vi "Module Execution Main.vi"() -> ()   [LabVIEW 2013, in "module execution process.lvlib"]
uses:
  module execution process.lvlib
  SubVIs/queue name.ctl
  SubVIs/command commands to rtexe process.ctl
  <vilib>/NI/Module Execution Interface/Engine Runtime/Engine Runtime Interface.lvclass
  <vilib>/NI/Configuration Framework/class discovery singleton/class discovery singleton methods.ctl
  <vilib>/NI/Tag Bus Data Framework/Framework Configuration Classes/target runtime/PL_Target Runtime.lvclass
  SubVIs/engine status data.ctl
  <vilib>/NI/Module Execution Interface/Engine Runtime/Execution States.ctl
  <vilib>/NI/AMC/Read Termination Message.vi
  <vilib>/NI/AMC/Create Single Message.vi
  <vilib>/NI/AMC/Globals.vi
  <vilib>/NI/Module Execution Interface/Engine Configuration/engine configuration.lvclass
  <vilib>/NI/Tag Bus Module Framework/module configuration/TBM module configuration.lvclass
  <vilib>/NI/Tag Bus Module Framework/runtime/TBM module execution interface.lvclass
  <vilib>/nisyscfg/nisyscfg.lvlib
  <vilib>/NI/Tag Bus Data Framework/Framework Configuration Classes/platypus configuration/PLConfigurationSerializer.lvlib
  <vilib>/NI/Configuration Framework/class discovery singleton/class discovery singleton.lvlib
  <vilib>/NI/AMC/AMC.lvlib
  <vilib>/NI/Configuration Framework/tree serializer/NISE_CEF_TreeSerializer.lvlib
  <vilib>/NI/Tag Bus Data Framework/Framework Configuration Classes/flattened data interface/PL_Serialization Interface.lvlib
panel:
  out "error out":errorcluster
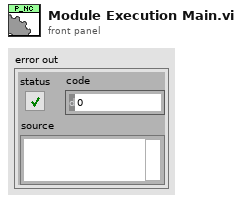
[diagram p1: front panel]
types:
  T1 = typedef "module execution process.lvlib/command commands to rtexe process.ctl" = enum16{"Initialize", "Load from File", "Load from String", "Open All Engines", "Open Single Engine", "Initialize All Engines", "Initialize Single Engine", "Start All", "Start Single", "Pause All", "Pause Single", "Stop All", "Stop Single", "Close All", "Close Single", "Set Safe State All", "Set Safe State Single", "Get Status", "Exit", "Error", "Add Search Paths"}
  T2 = typedef "module execution process.lvlib/queue name.ctl" = enum16{"TOrtmainexec", "FROMrtmainexec"}
  T3 = typedef "AMC.lvlib/Message Queue.ctl" = refnum<queue>
  T4 = typedef "class discovery singleton.lvlib/class discovery singleton methods.ctl" = enum16{"add search paths", "load class by name", "list available classes", "get class path"}
  T5 = typedef "module execution process.lvlib/engine status data.ctl" = cluster{"Name":string, "Engine State":T6, "Engine Error":errorcluster}
  T6 = typedef "Engine Runtime Interface.lvclass/Execution States.ctl" = enum16{"Initializing", "Paused (Initialized)", "Running", "Set Safe Outputs", "Uninitializing", "Stopped (Uninitialized)", "Error (Uninitialized)", "Safe State (Uninitialized)", "Closed"}
  T7 = typedef "module execution process.lvlib/configuration elements.ctl" = cluster{"Name":string, "opened?":bool, "configuration":T8, "engine":refnum<class "Engine Runtime Interface.lvclass">, "modules":refnum<class "TBM module execution interface.lvclass">[]}
  T8 = typedef "PLConfigurationSerializer.lvlib/engines cluster.ctl" = cluster{"engine configuration":refnum<class "engine configuration.lvclass">, "modules":refnum<class "TBM module configuration.lvclass">[]}
  T9 = typedef "NISE_CEF_TreeSerializer.lvlib/base file format.ctl" = cluster{"version":string, "data":string}
  T10 = typedef "NISE_CEF_TreeSerializer.lvlib/flat hierarchy.ctl" = cluster{"hierarchy structure":T11, "instance data":T13[]}
  T11 = typedef "NISE_CEF_TreeSerializer.lvlib/full hierarchy.ctl" = cluster{"root":string, "hierarchy":T12[]}
  T12 = typedef "NISE_CEF_TreeSerializer.lvlib/hierarchy element.ctl" = cluster{"current node":string, "children":string[]}
  T13 = typedef "NISE_CEF_TreeSerializer.lvlib/instance data.ctl" = cluster{"ID":string, "Alias":string, "class":string, "version":string, "data":string}
  T14 = typedef "PLConfigurationSerializer.lvlib/targets cluster.ctl" = cluster{"Target Configuration":refnum<class "PL_Target Configuration.lvclass">, "engines":T8[]}
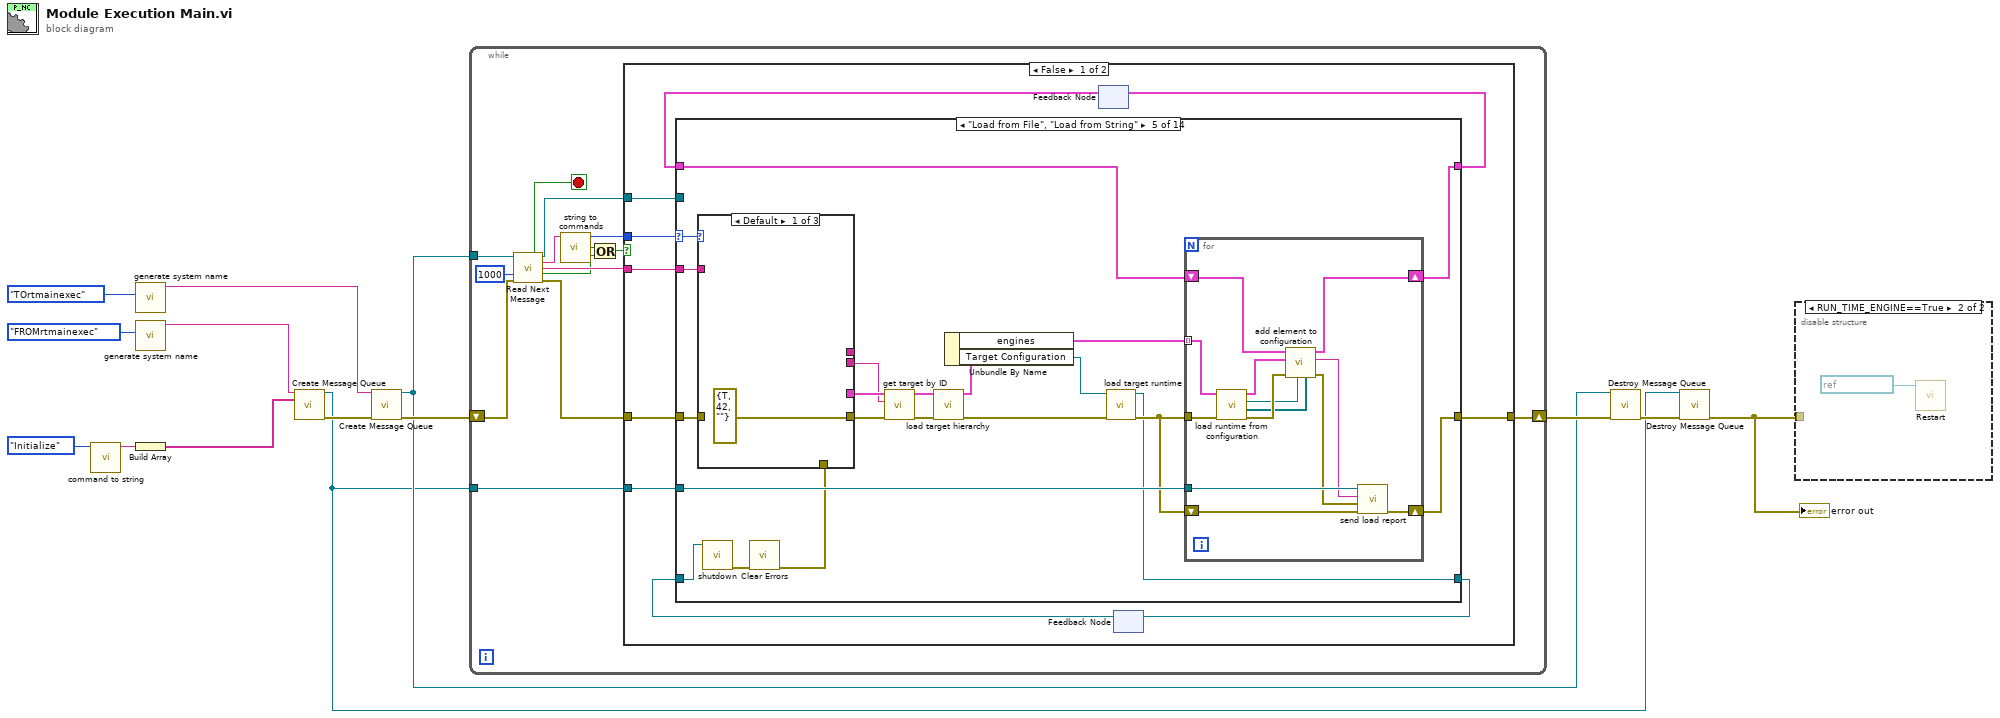
[diagram p0: block diagram]
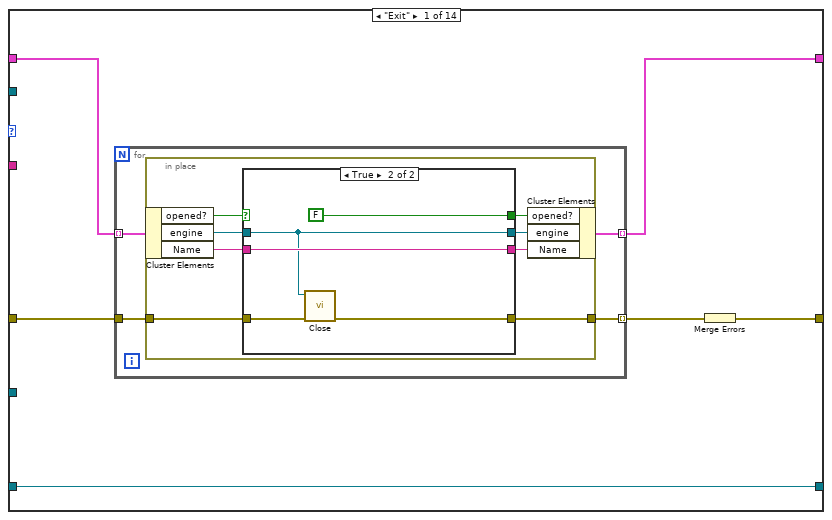
[diagram p3: hidden frame]
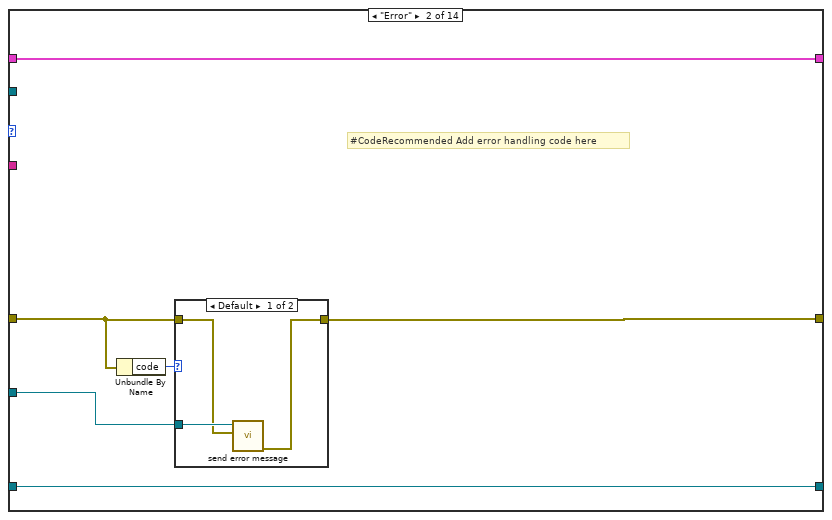
[diagram p5: hidden frame]
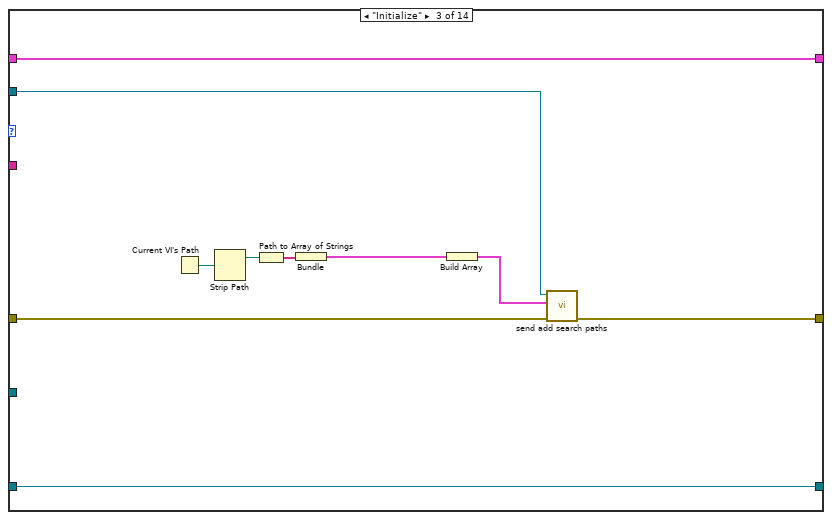
[diagram p7: hidden frame]
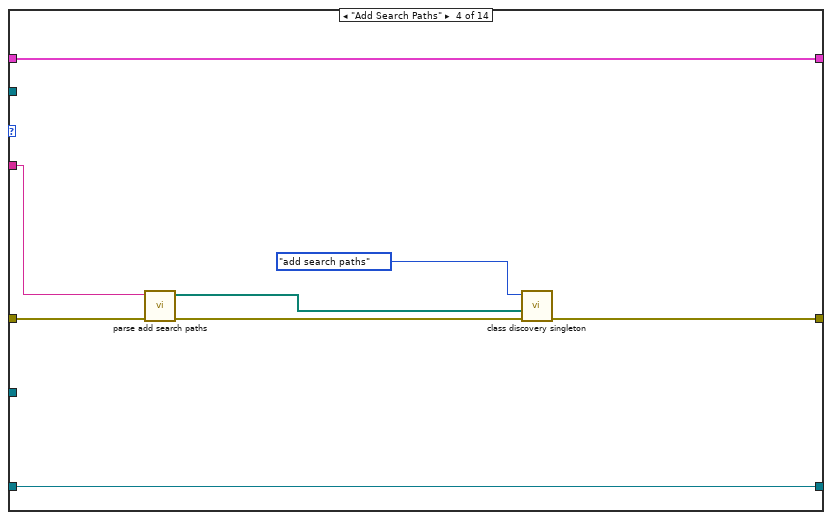
[diagram p8: hidden frame]
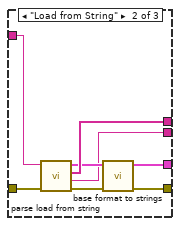
[diagram p9: hidden frame]
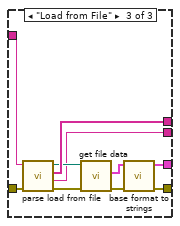
[diagram p10: hidden frame]
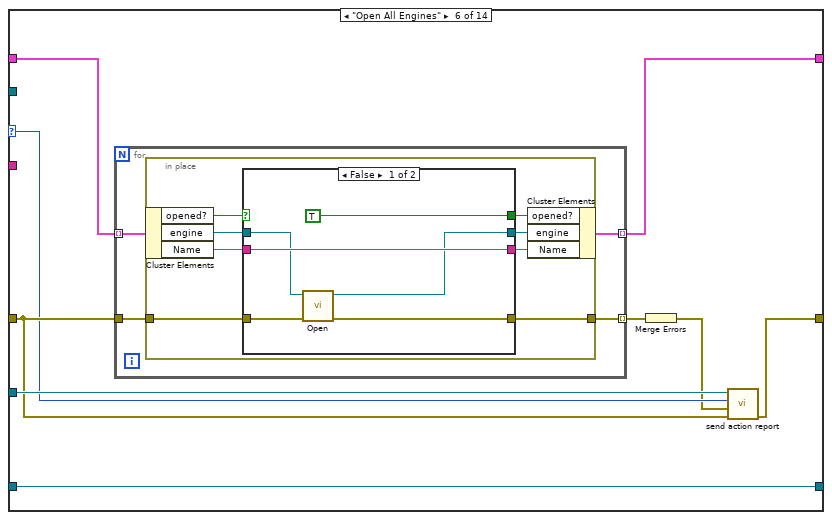
[diagram p11: hidden frame]
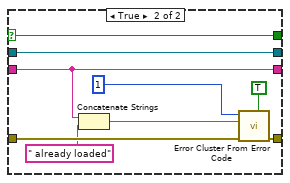
[diagram p12: hidden frame]
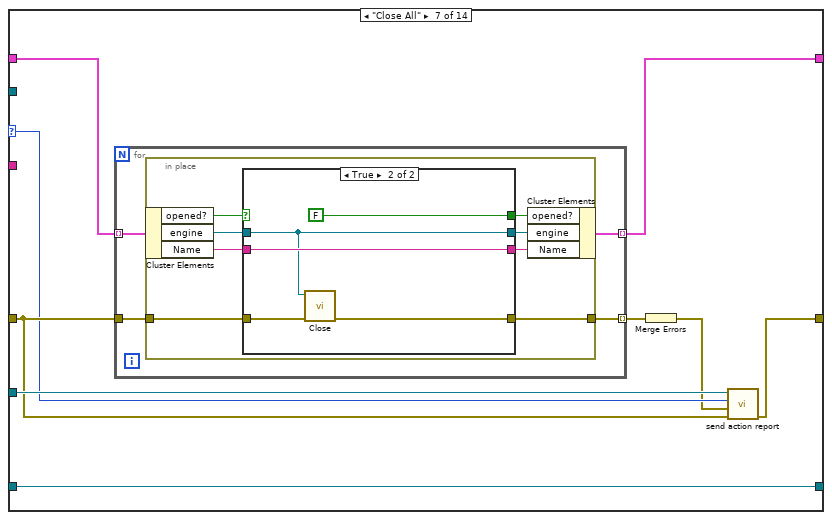
[diagram p13: hidden frame]
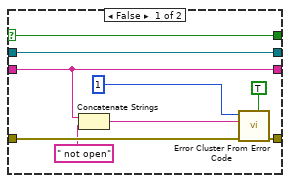
[diagram p14: hidden frame]
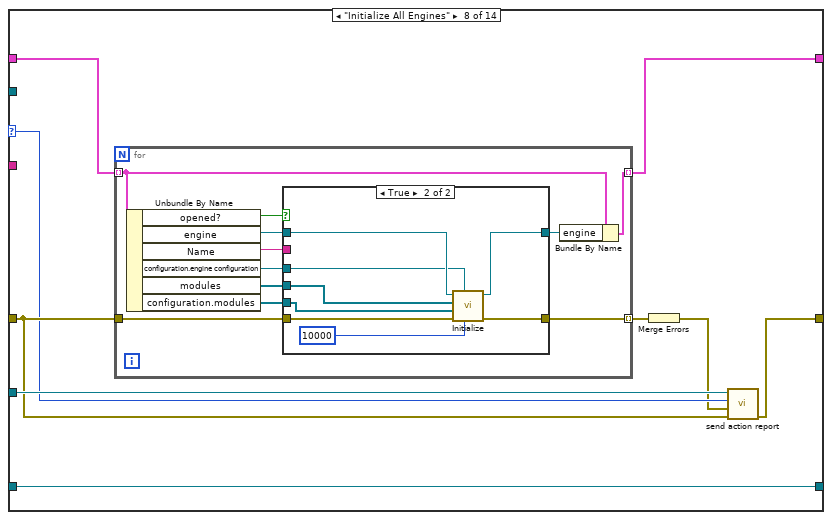
[diagram p15: hidden frame]
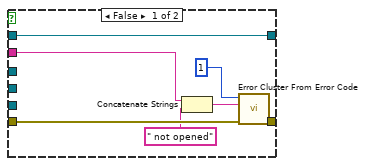
[diagram p16: hidden frame]
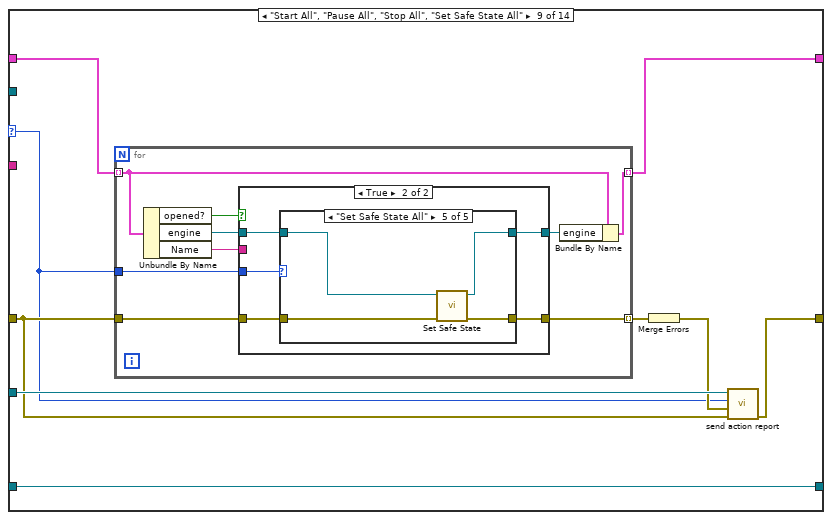
[diagram p17: hidden frame]
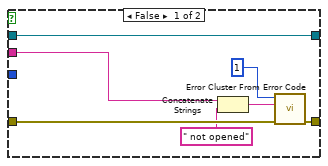
[diagram p18: hidden frame]
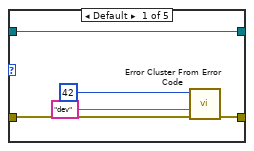
[diagram p19: hidden frame]
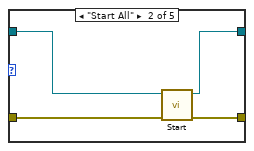
[diagram p20: hidden frame]
diagram:
  n1 = call "command to string.vi"("commands"=command_commands_to_rtexe_process."Initialize") -> ("command string"=w6:string)  [unwired: 10 in]
  n2 = call "generate system name.vi"("queue"=queue_name."TOrtmainexec") -> ("queue name"=w11:string)  [unwired: 10 in]
  n3 = call "generate system name.vi"("queue"=queue_name."FROMrtmainexec") -> ("queue name"=w13:string)  [unwired: 10 in]
  n4 = Build Array(w6) -> (w5:string[])
  n5 = call <vilib>:"Create Message Queue.vi"("message queue name"=w13, "initial message names"=w5) -> ("message queue out"=w1:T3, "error out"=w12:errorcluster)  [unwired: 12 in]
  n6 = call <vilib>:"Create Message Queue.vi"("message queue name"=w11, "error in"=w12) -> ("message queue out"=w2:T3, "error out"=w10:errorcluster)  [unwired: 12 in]
  n7 = while {
    tunnel: w2 -> [w26]
    shift-right: [w28] -> w14
    shift-left: w10 -> [w23]
    tunnel: w1 -> [w27]
    stop <- w25 stop-if-true
    n8 = call <vilib>:"Read Next Message.vi"("message queue in"=w26, "timeout (1 ms)"=1000, "error in"=w23) -> ("exit process?"=w25:bool, "message queue out"=w15:T3, "message name"=w20:string, "message value"=w24:string, "timed out?"=w18:bool, "error out"=w22:errorcluster)  [unwired: 5 in, 2 out]
    n9 = call "string to commands.vi"("command string"=w20) -> ("invalid"=w19:bool, "commands"=w16:T1)  [unwired: 9 in]
    n10 = Or(x=w19, y=w18) -> (x .or. y?=w17:bool)
    n11 = case shown="False" w17 {
      tunnel: w24 -> [w38 _]
      tunnel: [w37 w573] -> w28
      tunnel: w27 -> [w36 _]
      tunnel: w22 -> [w35 w573]
      tunnel: w16 -> [w34 _]
      tunnel: w15 -> [w33 _]
      frame False {
        n12 = feedback #1() -> (w31:T7[])  [unwired: 1 in]
        n13 = feedback #2() -> (w29:refnum<class "PL_Target Runtime.lvclass">)  [unwired: 1 in]
        n14 = case shown="\"Load from File\", \"Load from String\"" w34 {
          selector: w34 -> [_ _ _ _ w111 w148 w184 w219 w253 w313 w372 w430 w476 _]
          tunnel: w38 -> [_ _ _ w86 w113 _ _ _ _ w310 w369 w427 w483 _]
          tunnel: [w43 w71 w84 w92 w110 w153 w189 w224 w259 w316 w375 w433 w488 w549] -> w32
          tunnel: w31 -> [w44 w71 w84 w92 w109 w154 w190 w225 w260 w317 w376 w434 w489 w550]
          tunnel: [w40 w68 w82 w90 w108 w150 w186 w221 w256 w314 w373 w431 w486 w547] -> w37
          tunnel: w35 -> [w42 w69 w83 w89 w112 w151 w187 w222 w257 w312 w371 w429 w485 w548]
          tunnel: w36 -> [_ w67 _ _ w107 w152 w188 w223 w258 w315 w374 w432 w487 w546]
          tunnel: w33 -> [_ _ w81 _ _ _ _ _ _ _ _ _ _ _]
          tunnel: [w39 w66 w75 w85 w96 w146 w182 w217 w252 w303 w362 w420 w475 w544] -> w30
          tunnel: w29 -> [w39 w66 w75 w85 w95 w146 w182 w217 w252 w303 w362 w420 w475 w544]
          frame "Exit" {
            n15 = for {
              tunnel: w44 -> [w48] mode=indexing
              tunnel: [w47] -> w43 mode=indexing
              tunnel: w42 -> [w46]
              tunnel: [w45] -> w41 mode=indexing
              n16 = in-place {
                in-place-border: w46 -> [w53]
                in-place-border: [w52] -> w45
                n17 = in-place-cluster #3(w48) -> ("opened?"=w56:bool, "engine"=w55:refnum<class "Engine Runtime Interface.lvclass">, "Name"=w51:string)
                n18 = case shown="True" w56 {
                  selector: w56 -> [w57 _]
                  tunnel: w55 -> [w60 w61]
                  tunnel: [w60 w61] -> w54
                  tunnel: w53 -> [w59 w63]
                  tunnel: [w59 w62] -> w52
                  tunnel: w51 -> [w58 w65]
                  tunnel: [w58 w65] -> w50
                  tunnel: [w57 FALSE ("opened?")] -> w49
                  frame False {
                  }
                  frame True {
                    n19 = call-dynamic "Close.vi"("error in"=w63, "Engine Runtime Interface in"=w61) -> ("error out"=w62:errorcluster)  [unwired: 9 in]
                  }
                }
                n20 = in-place-cluster #3("opened?"=w49, "engine"=w54, "Name"=w50) -> (w47:T7)
              }
            }
            n21 = Merge Errors(w41) -> (w40:errorcluster)
          }
          frame "Error" {
            # "#CodeRecommended Add error handling code here"
            n22 = Unbundle By Name(w69) -> ("code"=w70:i32)
            n23 = case shown="Default" w70 {
              tunnel: w69 -> [w72 _]
              tunnel: [w73 _] -> w68
              tunnel: w67 -> [w74 _]
              frame Default {
                n24 = call "send error message.vi"("error to send"=w72, "message queue in"=w74) -> ("error out"=w73:errorcluster)  [unwired: 8 in, 1 out]
              }
              frame 538255 {
                # "Ignore this timeout error for now."
              }
            }
          }
          frame "Initialize" {
            n25 = Current VI's Path() -> (path=w80:path)
            n26 = Strip Path(path=w80) -> (stripped path=w79:path)  [unwired: 1 out]
            n27 = Path to Array of Strings(0:w79) -> (2:w78:string[])  [unwired: 1 out]
            n28 = Bundle("array of strings"=w78) -> (w77:cluster{"array of strings":string[]})  [unwired: 1 in]
            n29 = Build Array(w77) -> (w76:cluster{"array of strings":string[]}[])
            n30 = call "send add search paths.vi"("error in"=w83, "search paths"=w76, "message queue in"=w81) -> ("error out"=w82:errorcluster)  [unwired: 7 in, 1 out]
          }
          frame "Add Search Paths" {
            n31 = call "parse add search paths.vi"("error in"=w89, "message data"=w86) -> ("error out"=w88:errorcluster, "paths"=w87:path[])  [unwired: 8 in]
            n32 = call <vilib>:"class discovery singleton.vi"("error in"=w88, "Plugin Search Paths"=w87, "method"=class_discovery_singleton_methods."add search paths") -> ("error out"=w90:errorcluster)  [unwired: 5 in, 3 out]
          }
          frame "Load from File", "Load from String" {
            n33 = call-dynamic "shutdown.vi"("Target Runtime in"=w95) -> ("error out"=w94:errorcluster)  [unwired: 10 in]
            n34 = call <vilib>:"Clear Errors.vi"("error in (no error)"=w94) -> ("error out"=w93:errorcluster)  [unwired: 6 in]
            n35 = case shown="Default" w111 {
              tunnel: w113 -> [_ w134 w144]
              tunnel: w112 -> [_ w135 w145]
              tunnel: [errorcluster {"status"=TRUE, "code"=42, "source"=""} ("error out") w131 w138] -> w106
              tunnel: [_ w133 w143] -> _
              tunnel: [_ w132 w137] -> w105
              tunnel: [_ w128 w136] -> w104
              tunnel: w93 -> [_ _ _]
              frame Default {
              }
              frame "Load from String" {
                n36 = call "parse load from string.vi"("error in"=w135, "message data"=w134) -> ("error out"=w129:errorcluster, "target"=w128:string, "engines to load"=w133:string[], "data"=w130:T9)  [unwired: 6 in]
                n37 = call <vilib>:"base format to strings.vi"("error in"=w129, "format"=w130) -> ("error out"=w131:errorcluster, "data"=w132:T10)  [unwired: 8 in]
              }
              frame "Load from File" {
                n38 = call "parse load from file.vi"("error in"=w145, "message data"=w144) -> ("error out"=w139:errorcluster, "target to load"=w136:string, "engines to load"=w143:string[], "path"=w140:path)  [unwired: 6 in]
                n39 = call <vilib>:"get file data.vi"("error in"=w139, "Path"=w140) -> ("error out"=w141:errorcluster, "format"=w142:T9)  [unwired: 8 in]
                n40 = call <vilib>:"base format to strings.vi"("error in"=w141, "format"=w142) -> ("error out"=w138:errorcluster, "data"=w137:T10)  [unwired: 8 in]
              }
            }
            n41 = call <vilib>:"get target by ID.vi"("error in"=w106, "UID"=w104, "full system"=w105) -> ("error out"=w103:errorcluster, "target hierarchy"=w102:T10)  [unwired: 7 in]
            n42 = call <vilib>:"load target hierarchy.vi"("error in"=w103, "target hierarchy"=w102) -> ("error out"=w99:errorcluster, "targets cluster out"=w101:T14)  [unwired: 8 in]
            n43 = Unbundle By Name(w101) -> ("engines"=w100:T8[], "Target Configuration"=w97:refnum<class "PL_Target Configuration.lvclass">)
            n44 = call <vilib>:"load target runtime.vi"("error in"=w99, "target configuration"=w97) -> ("error out"=w98:errorcluster, "target runtime"=w96:refnum<class "PL_Target Runtime.lvclass">)  [unwired: 8 in]
            n45 = for {
              tunnel: w100 -> [w125] mode=indexing
              tunnel: w98 -> [w126]
              shift-right: [w120] -> w110
              shift-left: w109 -> [w119]
              shift-right: [w116] -> w108
              shift-left: w98 -> [w117]
              tunnel: w107 -> [w118]
              n46 = call <vilib>:"load runtime from configuration.vi"("error in"=w126, "engine configuration in"=w125) -> ("error out"=w124:errorcluster, "Component Runtime Objects"=w121:refnum<class "TBM module execution interface.lvclass">[], "Engine Runtime Object"=w122:refnum<class "Engine Runtime Interface.lvclass">, "engine configuration out"=w123:T8)  [unwired: 6 in]
              n47 = call "add element to configuration.vi"("Component Runtime Objects"=w121, "Engine Runtime Object"=w122, "error in"=w124, "engine configuration out"=w123, "Configuration in"=w119) -> ("error out"=w114:errorcluster, "engine loaded"=w115:string, "Configuration out"=w120:T7[])  [unwired: 4 in]
              n48 = call "send load report.vi"("error in"=w117, "load error"=w114, "engine loaded"=w115, "message queue in"=w118) -> ("error out"=w116:errorcluster)  [unwired: 6 in, 1 out]
            }
          }
          frame "Open All Engines" {
            n49 = for {
              tunnel: w154 -> [w158] mode=indexing
              tunnel: [w157] -> w153 mode=indexing
              tunnel: w151 -> [w156]
              tunnel: [w155] -> w149 mode=indexing
              n50 = in-place {
                in-place-border: w156 -> [w163]
                in-place-border: [w162] -> w155
                n51 = in-place-cluster #4(w158) -> ("opened?"=w166:bool, "engine"=w165:refnum<class "Engine Runtime Interface.lvclass">, "Name"=w161:string)
                n52 = case shown="False" w166 {
                  selector: w166 -> [_ w173]
                  tunnel: w165 -> [w169 w181]
                  tunnel: [w168 w181] -> w164
                  tunnel: w163 -> [w172 w180]
                  tunnel: [w171 w179] -> w162
                  tunnel: w161 -> [w170 w174]
                  tunnel: [w170 w174] -> w160
                  tunnel: [TRUE ("opened?") w173] -> w159
                  frame False {
                    n53 = call-dynamic "Open.vi"("error in"=w172, "Engine Runtime Interface in"=w169) -> ("error out"=w171:errorcluster, "Engine Runtime Interface out"=w168:refnum<class "Engine Runtime Interface.lvclass">)  [unwired: 8 in]
                  }
                  frame True {
                    n54 = Concatenate Strings(w174, " already loaded" ("string")) -> (w176:string)
                    n55 = call <vilib>:"Error Cluster From Error Code.vi"("is warning? (False)"=TRUE, "error in (no error)"=w180, "error message (\"\")"=w176, "error code (0)"=1) -> ("error out"=w179:errorcluster)  [unwired: 5 in]
                  }
                }
                n56 = in-place-cluster #4("opened?"=w159, "engine"=w164, "Name"=w160) -> (w157:T7)
              }
            }
            n57 = Merge Errors(w149) -> (w147:errorcluster)
            n58 = call "send action report.vi"("error in"=w151, "command error"=w147, "commands"=w148, "message queue in"=w152) -> ("error out"=w150:errorcluster)  [unwired: 6 in, 1 out]
          }
          frame "Close All" {
            n59 = for {
              tunnel: w190 -> [w194] mode=indexing
              tunnel: [w193] -> w189 mode=indexing
              tunnel: w187 -> [w192]
              tunnel: [w191] -> w185 mode=indexing
              n60 = in-place {
                in-place-border: w192 -> [w199]
                in-place-border: [w198] -> w191
                n61 = in-place-cluster #5(w194) -> ("opened?"=w202:bool, "engine"=w201:refnum<class "Engine Runtime Interface.lvclass">, "Name"=w197:string)
                n62 = case shown="True" w202 {
                  selector: w202 -> [w203 _]
                  tunnel: w201 -> [w211 w212]
                  tunnel: [w211 w212] -> w200
                  tunnel: w199 -> [w210 w214]
                  tunnel: [w209 w213] -> w198
                  tunnel: w197 -> [w204 w216]
                  tunnel: [w204 w216] -> w196
                  tunnel: [w203 FALSE ("opened?")] -> w195
                  frame False {
                    n63 = Concatenate Strings(w204, " not open" ("string")) -> (w206:string)
                    n64 = call <vilib>:"Error Cluster From Error Code.vi"("is warning? (False)"=TRUE, "error in (no error)"=w210, "error message (\"\")"=w206, "error code (0)"=1) -> ("error out"=w209:errorcluster)  [unwired: 5 in]
                  }
                  frame True {
                    n65 = call-dynamic "Close.vi"("error in"=w214, "Engine Runtime Interface in"=w212) -> ("error out"=w213:errorcluster)  [unwired: 9 in]
                  }
                }
                n66 = in-place-cluster #5("opened?"=w195, "engine"=w200, "Name"=w196) -> (w193:T7)
              }
            }
            n67 = Merge Errors(w185) -> (w183:errorcluster)
            n68 = call "send action report.vi"("error in"=w187, "command error"=w183, "commands"=w184, "message queue in"=w188) -> ("error out"=w186:errorcluster)  [unwired: 6 in, 1 out]
          }
          frame "Initialize All Engines" {
            n69 = for {
              tunnel: w225 -> [w236] mode=indexing
              tunnel: [w235] -> w224 mode=indexing
              tunnel: w222 -> [w234]
              tunnel: [w233] -> w220 mode=indexing
              n70 = Unbundle By Name(w236) -> ("opened?"=w232:bool, "engine"=w231:refnum<class "Engine Runtime Interface.lvclass">, "Name"=w229:string, "configuration.engine configuration"=w228:refnum<class "engine configuration.lvclass">, "modules"=w227:refnum<class "TBM module execution interface.lvclass">[], "configuration.modules"=w226:refnum<class "TBM module configuration.lvclass">[])
              n71 = case shown="True" w232 {
                tunnel: w231 -> [w243 w248]
                tunnel: [w243 w249] -> w230
                tunnel: w234 -> [w242 w250]
                tunnel: [w241 w251] -> w233
                tunnel: w229 -> [w237 _]
                tunnel: w228 -> [_ w247]
                tunnel: w227 -> [_ w246]
                tunnel: w226 -> [_ w245]
                frame False {
                  n72 = Concatenate Strings(w237, " not opened" ("string")) -> (w239:string)
                  n73 = call <vilib>:"Error Cluster From Error Code.vi"("error in (no error)"=w242, "error message (\"\")"=w239, "error code (0)"=1) -> ("error out"=w241:errorcluster)  [unwired: 6 in]
                }
                frame True {
                  n74 = call-dynamic "Initialize.vi"("timeout in ms"=10000, "Engine Configuration"=w247, "error in"=w250, "module Configurations"=w245, "modules"=w246, "Engine Runtime Interface in"=w248) -> ("error out"=w251:errorcluster, "Engine Runtime Interface out"=w249:refnum<class "Engine Runtime Interface.lvclass">)  [unwired: 4 in]
                }
              }
              n75 = Bundle By Name(cluster=w236, "engine"=w230) -> (w235:T7)
            }
            n76 = Merge Errors(w220) -> (w218:errorcluster)
            n77 = call "send action report.vi"("error in"=w222, "command error"=w218, "commands"=w219, "message queue in"=w223) -> ("error out"=w221:errorcluster)  [unwired: 6 in, 1 out]
          }
          frame "Start All", "Pause All", "Stop All", "Set Safe State All" {
            n78 = for {
              tunnel: w260 -> [w269] mode=indexing
              tunnel: [w268] -> w259 mode=indexing
              tunnel: w257 -> [w267]
              tunnel: [w266] -> w255 mode=indexing
              tunnel: w253 -> [w261]
              n79 = Unbundle By Name(w269) -> ("opened?"=w265:bool, "engine"=w264:refnum<class "Engine Runtime Interface.lvclass">, "Name"=w262:string)
              n80 = case shown="True" w265 {
                tunnel: w264 -> [w276 w278]
                tunnel: [w276 w279] -> w263
                tunnel: w267 -> [w275 w281]
                tunnel: [w274 w280] -> w266
                tunnel: w262 -> [w270 _]
                tunnel: w261 -> [_ w277]
                frame False {
                  n81 = Concatenate Strings(w270, " not opened" ("string")) -> (w272:string)
                  n82 = call <vilib>:"Error Cluster From Error Code.vi"("error in (no error)"=w275, "error message (\"\")"=w272, "error code (0)"=1) -> ("error out"=w274:errorcluster)  [unwired: 6 in]
                }
                frame True {
                  n83 = case shown="\"Set Safe State All\"" w277 {
                    tunnel: w281 -> [w284 w290 w294 w298 w302]
                    tunnel: [w285 w289 w293 w297 w301] -> w280
                    tunnel: [w286 w288 w292 w295 w300] -> w279
                    tunnel: w278 -> [w286 w287 w291 w296 w299]
                    frame Default {
                      n84 = call <vilib>:"Error Cluster From Error Code.vi"("error in (no error)"=w284, "error message (\"\")"="dev" ("error message (\"\")"), "error code (0)"=42) -> ("error out"=w285:errorcluster)  [unwired: 6 in]
                    }
                    frame "Start All" {
                      n85 = call-dynamic "Start.vi"("error in"=w290, "Engine Runtime Interface in"=w287) -> ("error out"=w289:errorcluster, "Engine Runtime Interface out"=w288:refnum<class "Engine Runtime Interface.lvclass">)  [unwired: 8 in]
                    }
                    frame "Pause All" {
                      n86 = call-dynamic "Pause.vi"("error in"=w294, "Engine Runtime Interface in"=w291) -> ("error out"=w293:errorcluster, "Engine Runtime Interface out"=w292:refnum<class "Engine Runtime Interface.lvclass">)  [unwired: 8 in]
                    }
                    frame "Stop All" {
                      n87 = call-dynamic "Stop.vi"("error in"=w298, "Engine Runtime Interface in"=w296) -> ("error out"=w297:errorcluster, "Engine Runtime Interface out"=w295:refnum<class "Engine Runtime Interface.lvclass">)  [unwired: 8 in]
                    }
                    frame "Set Safe State All" {
                      n88 = call-dynamic "Set Safe State.vi"("error in"=w302, "Engine Runtime Interface in"=w299) -> ("error out"=w301:errorcluster, "Engine Runtime Interface out"=w300:refnum<class "Engine Runtime Interface.lvclass">)  [unwired: 8 in]
                    }
                  }
                }
              }
              n89 = Bundle By Name(cluster=w269, "engine"=w263) -> (w268:T7)
            }
            n90 = Merge Errors(w255) -> (w254:errorcluster)
            n91 = call "send action report.vi"("error in"=w257, "command error"=w254, "commands"=w253, "message queue in"=w258) -> ("error out"=w256:errorcluster)  [unwired: 6 in, 1 out]
          }
          frame "Open Single Engine" {
            n92 = call "parse single action command.vi"("error in"=w312, "message data"=w310) -> ("error out"=w311:errorcluster, "engine name"=w309:string)  [unwired: 8 in]
            n93 = for {
              tunnel: w317 -> [w324] mode=indexing
              tunnel: [w323] -> w316 mode=indexing
              tunnel: w309 -> [w320]
              tunnel: [w319] -> w308 mode=indexing
              tunnel: w311 -> [w322]
              tunnel: [w321] -> w306
              stop <- w318 stop-if-true
              n94 = in-place {
                in-place-border: w322 -> [w331]
                in-place-border: [w330] -> w321
                in-place-border: w320 -> [w327]
                in-place-border: [w325] -> w319
                in-place-border: [w325] -> w318
                n95 = in-place-cluster #6(w324) -> ("opened?"=w334:bool, "engine"=w333:refnum<class "Engine Runtime Interface.lvclass">, "Name"=w326:string)
                n96 = Equal?(x=w326, y=w327) -> (x = y?=w325:bool)
                n97 = case shown="True" w325 {
                  tunnel: w334 -> [w338 w346]
                  tunnel: w333 -> [w337 w345]
                  tunnel: [w337 w344] -> w332
                  tunnel: w331 -> [w335 w343]
                  tunnel: [w335 w342] -> w330
                  tunnel: [w336 w341] -> w329
                  tunnel: [w338 w340] -> w328
                  tunnel: w326 -> [w336 w339]
                  frame False {
                  }
                  frame True {
                    n98 = case shown="False" w346 {
                      selector: w346 -> [_ w353]
                      tunnel: w345 -> [w349 w361]
                      tunnel: [w348 w361] -> w344
                      tunnel: w343 -> [w352 w360]
                      tunnel: [w351 w359] -> w342
                      tunnel: w339 -> [w350 w354]
                      tunnel: [w350 w354] -> w341
                      tunnel: [TRUE ("opened?") w353] -> w340
                      frame False {
                        n99 = call-dynamic "Open.vi"("error in"=w352, "Engine Runtime Interface in"=w349) -> ("error out"=w351:errorcluster, "Engine Runtime Interface out"=w348:refnum<class "Engine Runtime Interface.lvclass">)  [unwired: 8 in]
                      }
                      frame True {
                        n100 = Concatenate Strings(w354, " already loaded" ("string")) -> (w356:string)
                        n101 = call <vilib>:"Error Cluster From Error Code.vi"("is warning? (False)"=TRUE, "error in (no error)"=w360, "error message (\"\")"=w356, "error code (0)"=1) -> ("error out"=w359:errorcluster)  [unwired: 5 in]
                      }
                    }
                  }
                }
                n102 = in-place-cluster #6("opened?"=w328, "engine"=w332, "Name"=w329) -> (w323:T7)
              }
            }
            n103 = Or Array Elements(Boolean array=w308) -> (logical OR=w307:bool)
            n104 = Select(t=w306, s=w307, f=errorcluster {"status"=TRUE, "code"=1, "source"="Not found"}) -> (s? t:f=w305:errorcluster)
            n105 = call "send action report.vi"("error in"=w311, "command error"=w305, "commands"=w313, "message queue in"=w315) -> ("error out"=w314:errorcluster)  [unwired: 6 in, 1 out]
          }
          frame "Close Single" {
            n106 = call "parse single action command.vi"("error in"=w371, "message data"=w369) -> ("error out"=w370:errorcluster, "engine name"=w368:string)  [unwired: 8 in]
            n107 = for {
              tunnel: w376 -> [w383] mode=indexing
              tunnel: [w382] -> w375 mode=indexing
              tunnel: w368 -> [w379]
              tunnel: [w378] -> w367 mode=indexing
              tunnel: w370 -> [w381]
              tunnel: [w380] -> w365
              stop <- w377 stop-if-true
              n108 = in-place {
                in-place-border: w381 -> [w390]
                in-place-border: [w389] -> w380
                in-place-border: w379 -> [w386]
                in-place-border: [w384] -> w378
                in-place-border: [w384] -> w377
                n109 = in-place-cluster #7(w383) -> ("opened?"=w393:bool, "engine"=w392:refnum<class "Engine Runtime Interface.lvclass">, "Name"=w385:string)
                n110 = Equal?(x=w385, y=w386) -> (x = y?=w384:bool)
                n111 = case shown="True" w384 {
                  tunnel: w393 -> [w397 w405]
                  tunnel: w392 -> [w396 w404]
                  tunnel: [w396 w403] -> w391
                  tunnel: w390 -> [w394 w402]
                  tunnel: [w394 w401] -> w389
                  tunnel: [w395 w400] -> w388
                  tunnel: [w397 w399] -> w387
                  tunnel: w385 -> [w395 w398]
                  frame False {
                  }
                  frame True {
                    n112 = case shown="True" w405 {
                      selector: w405 -> [w406 _]
                      tunnel: w404 -> [w414 w415]
                      tunnel: [w414 w415] -> w403
                      tunnel: w402 -> [w413 w416]
                      tunnel: [w412 w417] -> w401
                      tunnel: w398 -> [w407 w419]
                      tunnel: [w407 w419] -> w400
                      tunnel: [w406 FALSE ("opened?")] -> w399
                      frame False {
                        n113 = Concatenate Strings(w407, " not opened" ("string")) -> (w409:string)
                        n114 = call <vilib>:"Error Cluster From Error Code.vi"("is warning? (False)"=TRUE, "error in (no error)"=w413, "error message (\"\")"=w409, "error code (0)"=1) -> ("error out"=w412:errorcluster)  [unwired: 5 in]
                      }
                      frame True {
                        n115 = call-dynamic "Close.vi"("error in"=w416, "Engine Runtime Interface in"=w415) -> ("error out"=w417:errorcluster)  [unwired: 9 in]
                      }
                    }
                  }
                }
                n116 = in-place-cluster #7("opened?"=w387, "engine"=w391, "Name"=w388) -> (w382:T7)
              }
            }
            n117 = Or Array Elements(Boolean array=w367) -> (logical OR=w366:bool)
            n118 = Select(t=w365, s=w366, f=errorcluster {"status"=TRUE, "code"=1, "source"="Not found"}) -> (s? t:f=w364:errorcluster)
            n119 = call "send action report.vi"("error in"=w370, "command error"=w364, "commands"=w372, "message queue in"=w374) -> ("error out"=w373:errorcluster)  [unwired: 6 in, 1 out]
          }
          frame "Initialize Single Engine" {
            n120 = call "parse single action command.vi"("error in"=w429, "message data"=w427) -> ("error out"=w428:errorcluster, "engine name"=w426:string)  [unwired: 8 in]
            n121 = for {
              tunnel: w434 -> [w447] mode=indexing
              tunnel: [w446] -> w433 mode=indexing
              tunnel: w426 -> [w443]
              tunnel: [w442] -> w425 mode=indexing
              tunnel: w428 -> [w445]
              tunnel: [w444] -> w423
              stop <- w442 stop-if-true
              n122 = Unbundle By Name(w447) -> ("configuration.engine configuration"=w435:refnum<class "engine configuration.lvclass">, "opened?"=w441:bool, "engine"=w440:refnum<class "Engine Runtime Interface.lvclass">, "modules"=w436:refnum<class "TBM module execution interface.lvclass">[], "configuration.modules"=w437:refnum<class "TBM module configuration.lvclass">[], "Name"=w438:string)
              n123 = Equal?(x=w438, y=w443) -> (x = y?=w442:bool)
              n124 = case shown="True" w442 {
                tunnel: w441 -> [_ w458]
                tunnel: w440 -> [w449 w457]
                tunnel: [w449 w456] -> w439
                tunnel: w445 -> [w448 w455]
                tunnel: [w448 w454] -> w444
                tunnel: w438 -> [_ w453]
                tunnel: w437 -> [_ w452]
                tunnel: w436 -> [_ w451]
                tunnel: w435 -> [_ w450]
                frame False {
                }
                frame True {
                  n125 = case shown="True" w458 {
                    tunnel: w457 -> [w466 w472]
                    tunnel: [w466 w471] -> w456
                    tunnel: w455 -> [w465 w473]
                    tunnel: [w464 w470] -> w454
                    tunnel: w453 -> [w459 _]
                    tunnel: w452 -> [_ w469]
                    tunnel: w451 -> [_ w468]
                    tunnel: w450 -> [_ w467]
                    frame False {
                      n126 = Concatenate Strings(w459, " not opened" ("string")) -> (w461:string)
                      n127 = call <vilib>:"Error Cluster From Error Code.vi"("is warning? (False)"=TRUE, "error in (no error)"=w465, "error message (\"\")"=w461, "error code (0)"=1) -> ("error out"=w464:errorcluster)  [unwired: 5 in]
                    }
                    frame True {
                      n128 = call-dynamic "Initialize.vi"("timeout in ms"=10000, "Engine Configuration"=w467, "error in"=w473, "module Configurations"=w469, "modules"=w468, "Engine Runtime Interface in"=w472) -> ("error out"=w470:errorcluster, "Engine Runtime Interface out"=w471:refnum<class "Engine Runtime Interface.lvclass">)  [unwired: 4 in]
                    }
                  }
                }
              }
              n129 = Bundle By Name(cluster=w447, "engine"=w439) -> (w446:T7)
            }
            n130 = Or Array Elements(Boolean array=w425) -> (logical OR=w424:bool)
            n131 = Select(t=w423, s=w424, f=errorcluster {"status"=TRUE, "code"=1, "source"="Not found"}) -> (s? t:f=w422:errorcluster)
            n132 = call "send action report.vi"("error in"=w428, "command error"=w422, "commands"=w430, "message queue in"=w432) -> ("error out"=w431:errorcluster)  [unwired: 6 in, 1 out]
          }
          frame "Start Single", "Pause Single", "Stop Single", "Set Safe State Single" {
            n133 = call "parse single action command.vi"("error in"=w485, "message data"=w483) -> ("error out"=w484:errorcluster, "engine name"=w482:string)  [unwired: 8 in]
            n134 = for {
              tunnel: w489 -> [w500] mode=indexing
              tunnel: [w499] -> w488 mode=indexing
              tunnel: w482 -> [w496]
              tunnel: [w495] -> w481 mode=indexing
              tunnel: w484 -> [w498]
              tunnel: [w497] -> w479
              tunnel: w476 -> [w490]
              stop <- w495 stop-if-true
              n135 = Unbundle By Name(w500) -> ("opened?"=w494:bool, "engine"=w493:refnum<class "Engine Runtime Interface.lvclass">, "Name"=w491:string)
              n136 = Equal?(x=w491, y=w496) -> (x = y?=w495:bool)
              n137 = case shown="True" w495 {
                tunnel: w494 -> [_ w509]
                tunnel: w493 -> [w502 w508]
                tunnel: [w502 w507] -> w492
                tunnel: w498 -> [w501 w506]
                tunnel: [w501 w505] -> w497
                tunnel: w491 -> [_ w504]
                tunnel: w490 -> [_ w503]
                frame False {
                }
                frame True {
                  n138 = case shown="True" w509 {
                    tunnel: w508 -> [w517 w520]
                    tunnel: [w517 w521] -> w507
                    tunnel: w506 -> [w516 w519]
                    tunnel: [w515 w522] -> w505
                    tunnel: w504 -> [w510 _]
                    tunnel: w503 -> [_ w518]
                    frame False {
                      n139 = Concatenate Strings(w510, " not opened" ("string")) -> (w512:string)
                      n140 = call <vilib>:"Error Cluster From Error Code.vi"("is warning? (False)"=TRUE, "error in (no error)"=w516, "error message (\"\")"=w512, "error code (0)"=1) -> ("error out"=w515:errorcluster)  [unwired: 5 in]
                    }
                    frame True {
                      n141 = case shown="\"Set Safe State Single\"" w518 {
                        tunnel: w519 -> [w525 w531 w535 w539 w543]
                        tunnel: [w526 w530 w534 w538 w542] -> w522
                        tunnel: [w527 w529 w533 w537 w540] -> w521
                        tunnel: w520 -> [w527 w528 w532 w536 w541]
                        frame Default {
                          n142 = call <vilib>:"Error Cluster From Error Code.vi"("error in (no error)"=w525, "error message (\"\")"="dev" ("error message (\"\")"), "error code (0)"=42) -> ("error out"=w526:errorcluster)  [unwired: 6 in]
                        }
                        frame "Start Single" {
                          n143 = call-dynamic "Start.vi"("error in"=w531, "Engine Runtime Interface in"=w528) -> ("error out"=w530:errorcluster, "Engine Runtime Interface out"=w529:refnum<class "Engine Runtime Interface.lvclass">)  [unwired: 8 in]
                        }
                        frame "Pause Single" {
                          n144 = call-dynamic "Pause.vi"("error in"=w535, "Engine Runtime Interface in"=w532) -> ("error out"=w534:errorcluster, "Engine Runtime Interface out"=w533:refnum<class "Engine Runtime Interface.lvclass">)  [unwired: 8 in]
                        }
                        frame "Set Safe State Single" {
                          n145 = call-dynamic "Set Safe State.vi"("error in"=w539, "Engine Runtime Interface in"=w536) -> ("error out"=w538:errorcluster, "Engine Runtime Interface out"=w537:refnum<class "Engine Runtime Interface.lvclass">)  [unwired: 8 in]
                        }
                        frame "Stop Single" {
                          n146 = call-dynamic "Stop.vi"("error in"=w543, "Engine Runtime Interface in"=w541) -> ("error out"=w542:errorcluster, "Engine Runtime Interface out"=w540:refnum<class "Engine Runtime Interface.lvclass">)  [unwired: 8 in]
                        }
                      }
                    }
                  }
                }
              }
              n147 = Bundle By Name(cluster=w500, "engine"=w492) -> (w499:T7)
            }
            n148 = Or Array Elements(Boolean array=w481) -> (logical OR=w480:bool)
            n149 = Select(t=w479, s=w480, f=errorcluster {"status"=TRUE, "code"=1, "source"="Not found"}) -> (s? t:f=w478:errorcluster)
            n150 = call "send action report.vi"("error in"=w484, "command error"=w478, "commands"=w476, "message queue in"=w487) -> ("error out"=w486:errorcluster)  [unwired: 6 in, 1 out]
          }
          frame "Get Status" {
            n151 = for {
              tunnel: w550 -> [w561] mode=indexing
              tunnel: [w560] -> w549 mode=indexing
              tunnel: w548 -> [w559]
              tunnel: [w555] -> w545 mode=indexing
              n152 = Unbundle By Name(w561) -> ("Name"=w551:string, "opened?"=w558:bool, "engine"=w557:refnum<class "Engine Runtime Interface.lvclass">)
              n153 = case shown="True" w558 {
                tunnel: w557 -> [w563 w570]
                tunnel: [w563 w567] -> w556
                tunnel: w559 -> [_ w572]
                tunnel: [Execution_States."Closed" ("Engine State") w568] -> w552
                tunnel: [_ w565] -> w553
                frame False {
                }
                frame True {
                  n154 = call-dynamic "Get State.vi"("error in"=w572, "Engine Runtime Interface in"=w570) -> ("error out"=w571:errorcluster, "Engine State"=w568:T6, "Engine Runtime Interface out"=w569:refnum<class "Engine Runtime Interface.lvclass">)  [unwired: 7 in]
                  n155 = call-dynamic "Read Buffered Error.vi"("error in"=w571, "Engine Runtime Interface in"=w569) -> ("error out"=w564:errorcluster, "Engine Error"=w566:errorcluster, "Engine Runtime Interface out"=w567:refnum<class "Engine Runtime Interface.lvclass">)  [unwired: 7 in]
                  n156 = Merge Errors(w566, w564) -> (w565:errorcluster)
                }
              }
              n157 = Bundle By Name(cluster=w561, "engine"=w556) -> (w560:T7)
              n158 = Bundle(cluster=T5 {"Name"="", "Engine State"=enum."Initializing", "Engine Error"={"status"=FALSE, "code"=0, "source"=""}}, "Name"=w551, "Engine State"=w552, "Engine Error"=w553) -> (w555:T5)
            }
            n159 = call "send engine statuses.vi"("error in"=w548, "statuses"=w545, "message queue in"=w546) -> ("error out"=w547:errorcluster)  [unwired: 7 in, 1 out]
          }
        }
        n160 = feedback-in #1(w32) -> ()
        n161 = feedback-in #2(w30) -> ()
      }
      frame True {
      }
    }
  }
  n162 = call <vilib>:"Destroy Message Queue.vi"("message queue in"=w2, "error in"=w14) -> ("error out"=w4:errorcluster)  [unwired: 11 in, 2 out]
  n163 = call <vilib>:"Destroy Message Queue.vi"("message queue in"=w1, "error in"=w4) -> ("error out"=w3:errorcluster)  [unwired: 11 in, 2 out]
  "error out" <- w3
  n164 = disable-structure shown="RUN_TIME_ENGINE==True" {
    disable-tunnel: w3 -> [_ _]
    frame condition #0 (active) {
    }
    frame condition #1 {
      n165 = call <vilib>:"Restart.vi"("Session in"=refnum<k21> "localhost" ("session in")) -> ()  [unwired: 8 in, 3 out]
    }
  }
